vi "Register Reflection Descriptors.vi"(8 "error in":errorcluster, 10 "reflector description strings":string[](array[string]), 11 "gRPCid in":T1) -> (0 "error out":errorcluster, 3 "gRPCid out":T1)   [LabVIEW 2019, in "grpc-lvsupport.lvlib"]
uses:
  grpc-lvsupport.lvlib
  Shared/grpcId.ctl
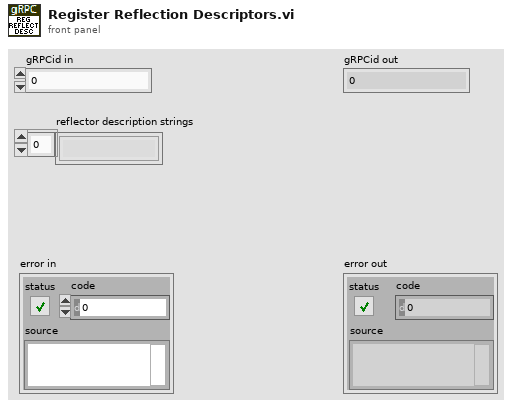
[diagram p1: front panel]
types:
  T1 = typedef "grpc-lvsupport.lvlib/grpcId.ctl" = u64
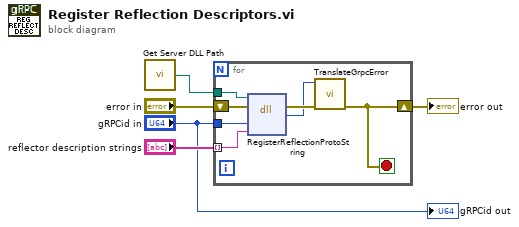
[diagram p0: block diagram]
diagram:
  n1 = call "Get Server DLL Path.vi"() -> ("server dll path"=w4:path)
  n2 = for {
    tunnel: w4 -> [w12]
    tunnel: "reflector description strings" -> [w11] mode=indexing
    shift-right: [w7] -> w5
    shift-left: "error in" -> [w10]
    tunnel: "gRPCid in" -> [w9]
    stop <- w7 stop-if-true
    n3 = dll-call lib="?" fn="RegisterReflectionProtoString"(path in=w12, error in=w10, "id"=w9, "serializedDescriptor"=w11) -> (error out=w8:errorcluster, "return type"=w6:i32)  [unwired: 3 in, 1 out]
    n4 = call "TranslateGrpcError.vi"("error in"=w8, "Error Code"=w6) -> ("error out"=w7:errorcluster)  [unwired: 9 in]
  }
  "error out" <- w5
  "gRPCid out" <- "gRPCid in"
